vi "主程序.vi"() -> ()   [LabVIEW 2012]
uses:
  <vilib>/Utility/miscctls.llb/LVRGBAColorTypeDef.ctl
  <vilib>/addons/control/pid/pid.llb/PID (DBL).vi
  <vilib>/addons/control/pid/NI_PID_pid.lvlib
  <vilib>/picture/3D Picture Control/NI_3D Picture Control.lvlib
panel:
  out "摆臂角度":dbl(graph)=-1.40625
  out "旋转臂角度":cluster{"旋转臂测量角度 3":dbl, dbl}(graph)={"旋转臂测量角度 3"=-61.25, -2.1437500000000003}
  out "输出电压":dbl(graph)=0.6637500000000003
  in  "输出电压1":dbl(graph)=0.6637500000000003
  out "三维图片":refnum<vi>(3d-picture)
  out "程序状态":bool=TRUE
  in  "继续按钮":bool
  in  "暂停按钮":bool
  out "摆臂角度输出 2":dbl=898.59375
  out "摆臂角度输出":dbl=178.59375
  out "摆臂角度1":dbl(graph)=-1.40625
  out "旋转臂角度1":cluster{"旋转臂测量角度 3":dbl, dbl}(graph)={"旋转臂测量角度 3"=-61.25, -2.1437500000000003}
  in  "副控制器PID参数":T1={"比例系数(Kc)"=0.9, "积分系数(Ti,min)"=0.0, "微分时间(Td/min)"=0.001}
  in  "主控制器PID参数":T1={"比例系数(Kc)"=0.035, "积分系数(Ti,min)"=0.0, "微分时间(Td/min)"=0.009}
  in  "?":bool=TRUE
  in  "副控制器设定值":dbl
  in  "K1":dbl=0.02
  in  "K2":dbl=-0.0
  in  "副控制器控制周期":u32=5
  out "output":dbl=-2.1437500000000003 format="%.2f"
  in  "停止":bool
  in  "主控制器控制周期":u32=15
  out "旋转臂测量角度 3":dbl=-61.25
  in  "主控制器设定值":dbl format="%.2f"
  # "一阶倒立摆串级PID控制\n测控技术与仪器                       1502班                                刘芳扬"
  # "副控制器系数"
  # "三维视图"
  # "测量显示"
  # "ms"
  # "控制方式"
  # "单回路"
  # "串级"
  # "主控制器系数"
  # "启停设置"
  # "ms"
  # "起摆系数"
  # "程序停止"
  # "程序暂停"
  # "程序继续"
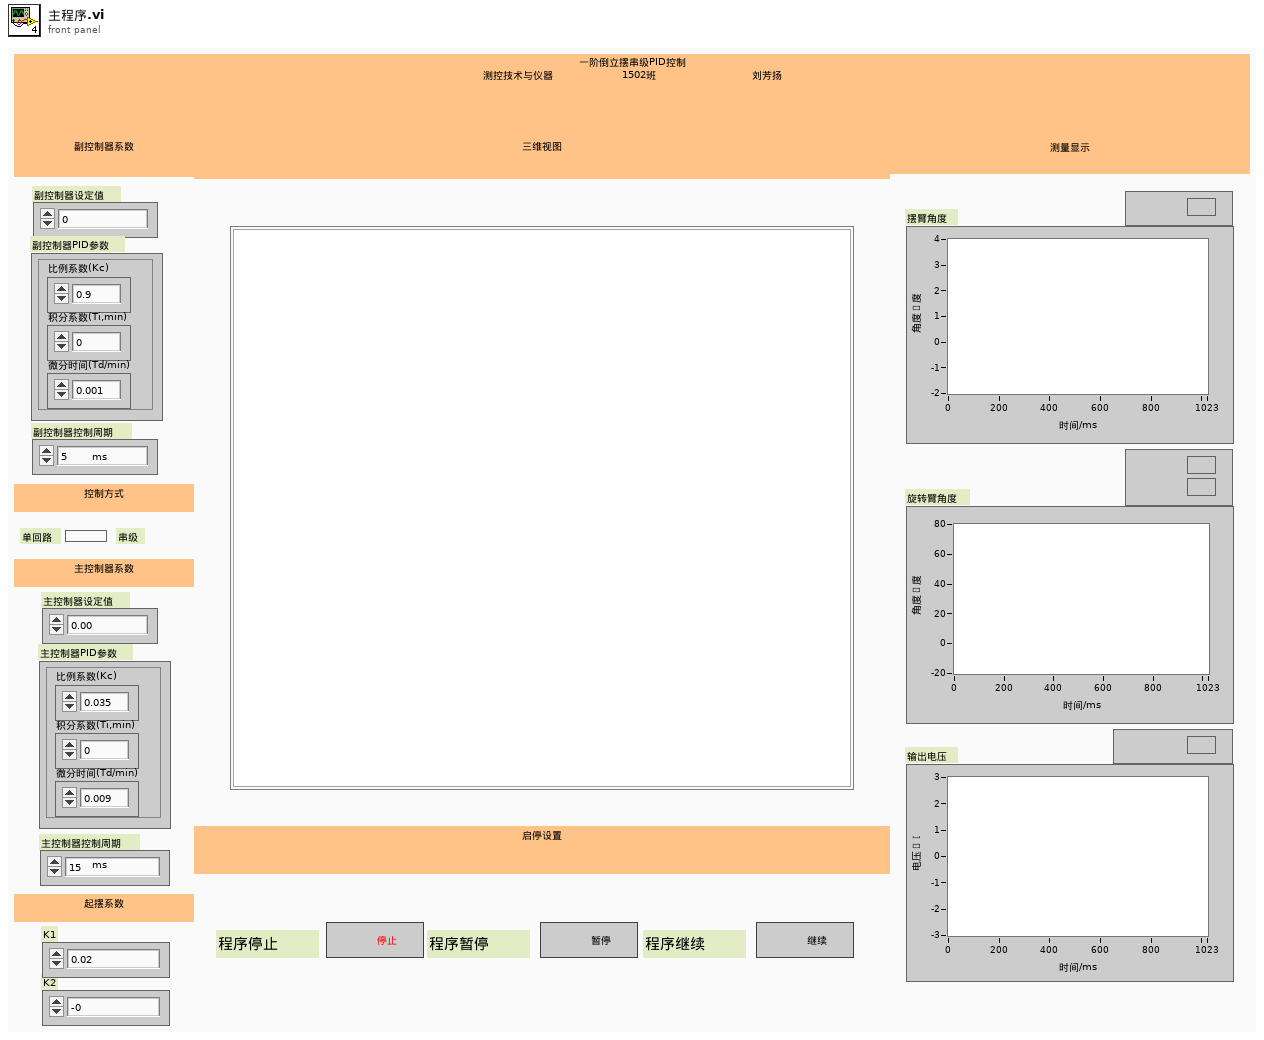
[diagram p1: front panel]
types:
  T1 = cluster{"比例系数(Kc)":dbl, "积分系数(Ti,min)":dbl, "微分时间(Td/min)":dbl}
  T2 = typedef "LVRGBAColorTypeDef.ctl" = cluster{"Red":sgl, "Green":sgl, "Blue":sgl, "Alpha":sgl}
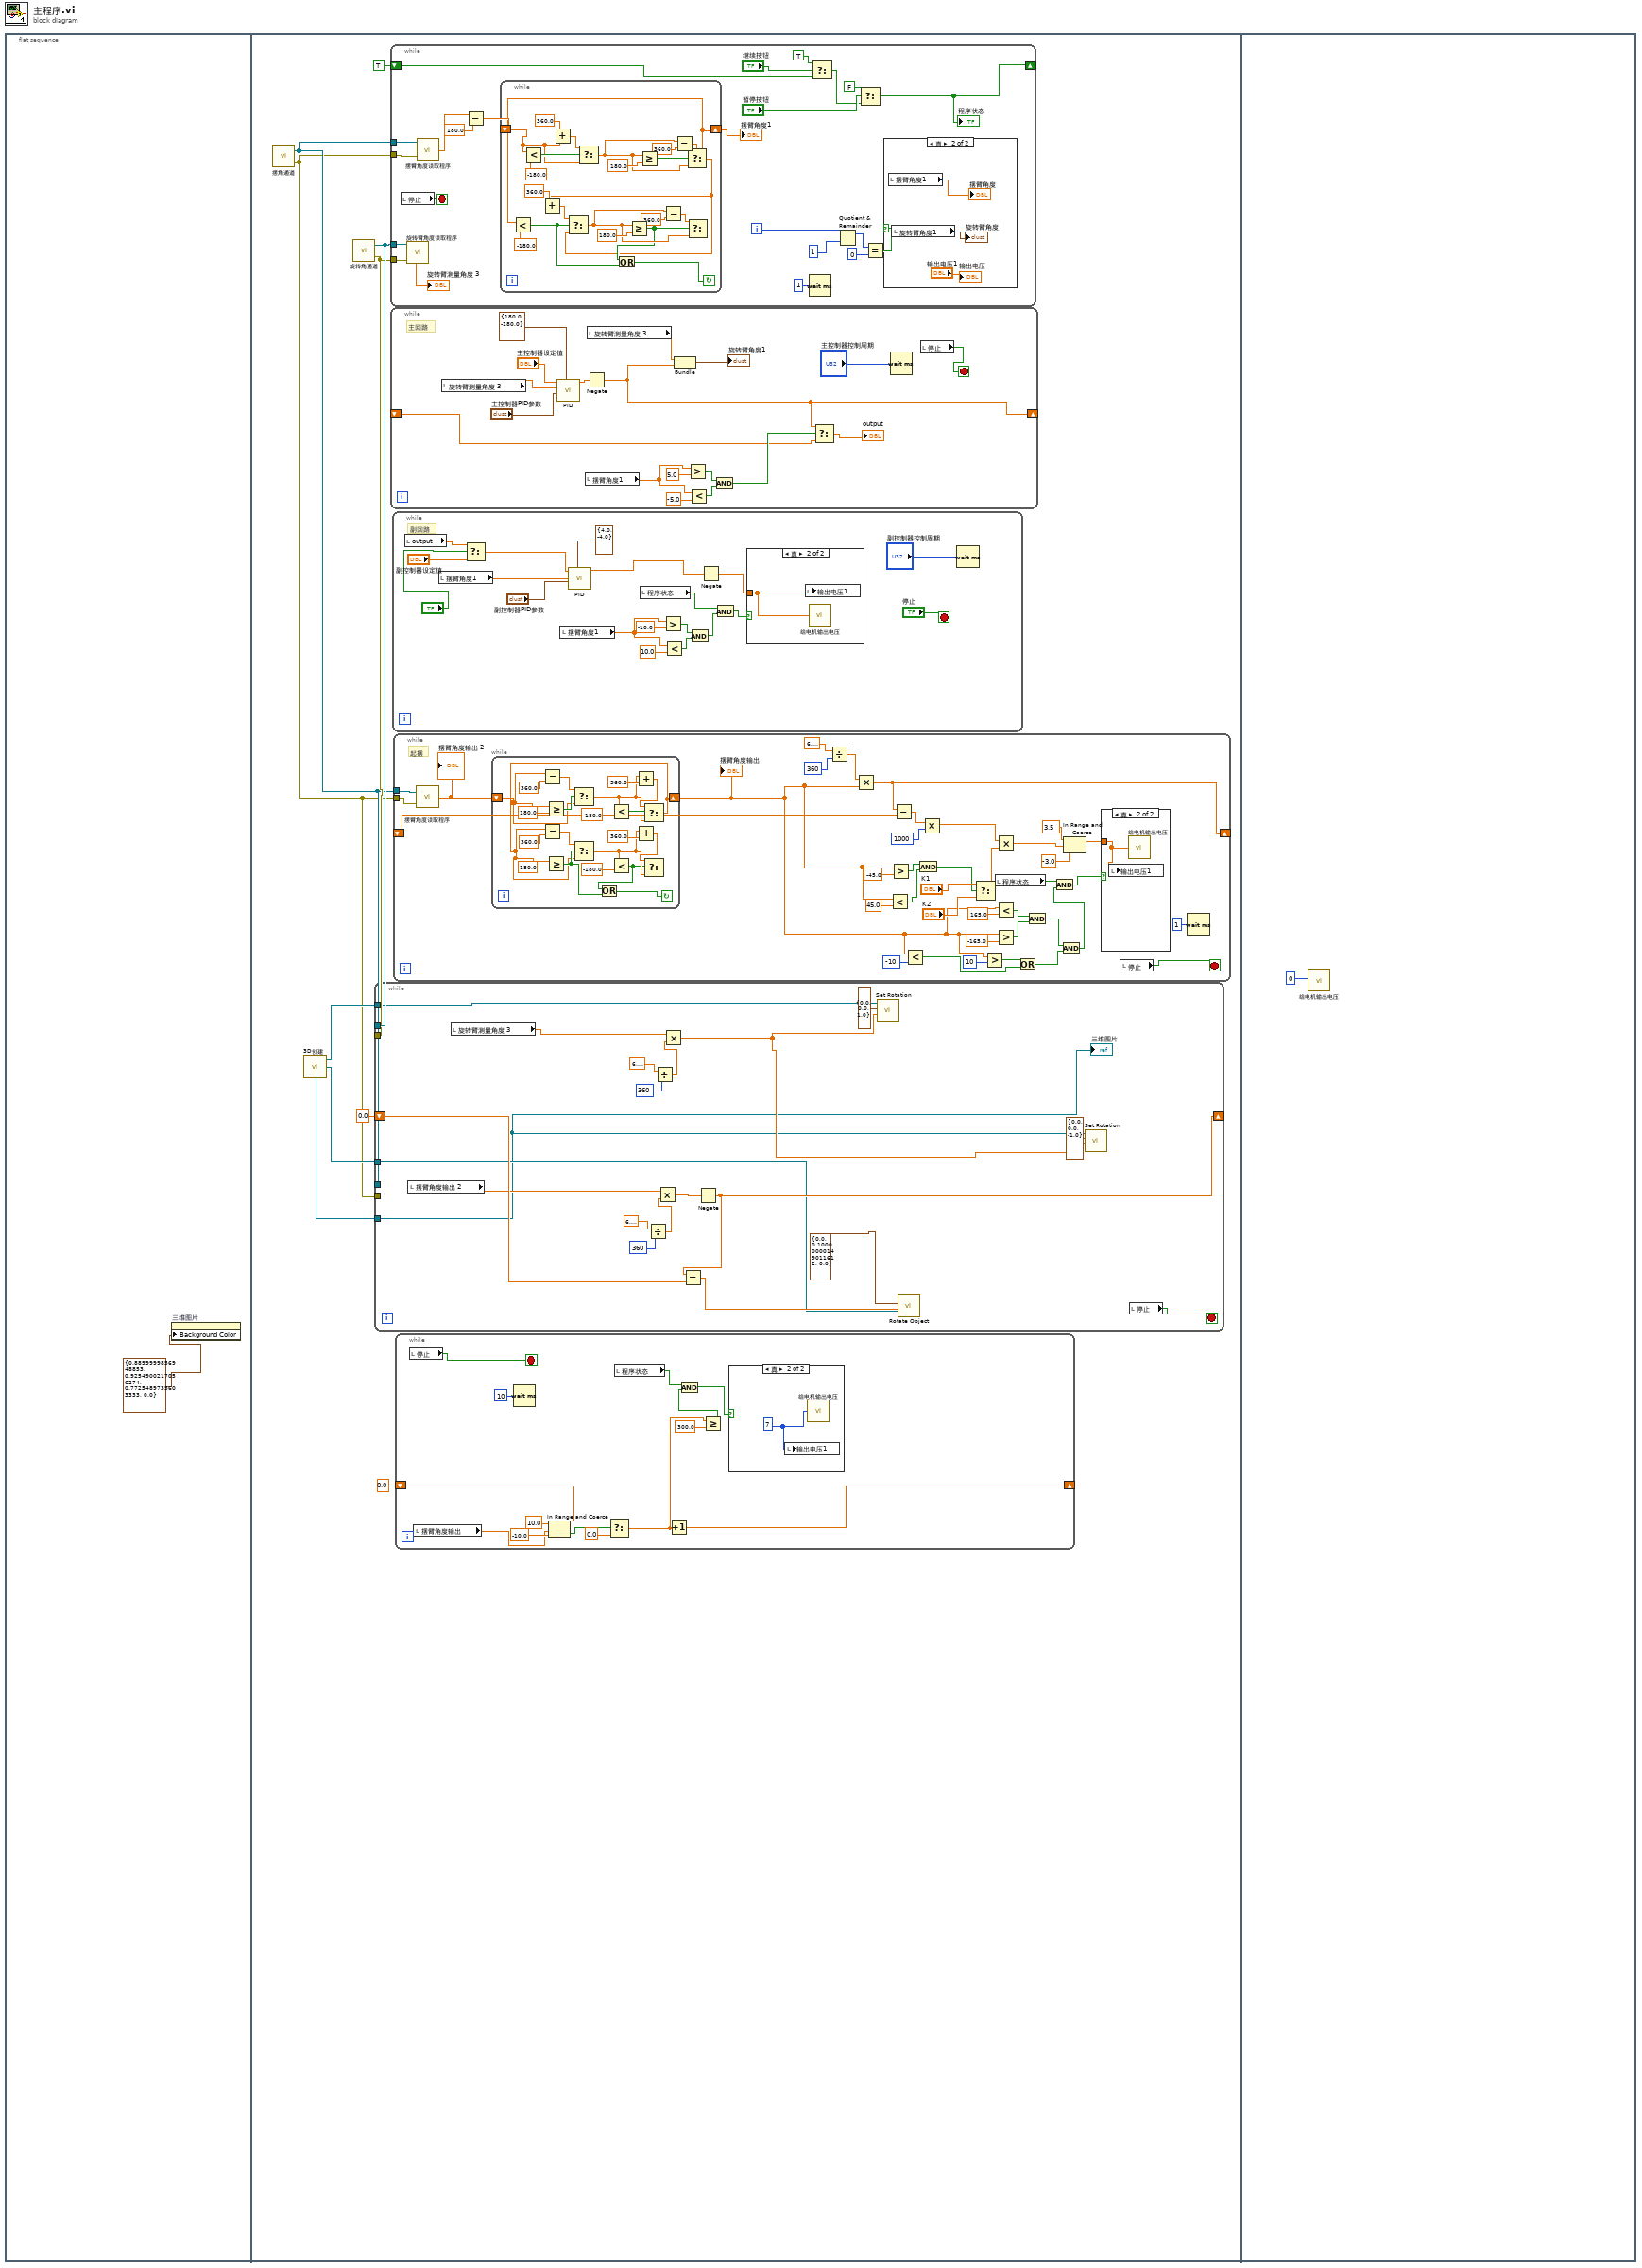
[diagram p0: block diagram]
diagram:
  n1 = flat-sequence {
    frame #0 {
      n2 = property on="三维图片" class="SceneGraphDisp (严格)"("Background Color"=T2 {"Red"=0.89, "Green"=0.92549, "Blue"=0.772549, "Alpha"=0.0} ("背景色")) -> ()  [unwired: 2 in, 2 out]
    }
    frame #1 {
      n3 = call "摆角通道.vi"() -> ("error out"=w5:errorcluster, "task out"=w6:refnum<k21>)  [unwired: 2 in]
      n4 = call "3D创建.vi"() -> ("旋转臂"=w9:refnum<vi>, "摆臂"=w10:refnum<vi>, "底座"=w11:refnum<vi>)
      n5 = call "旋转角通道.vi"() -> ("error out"=w7:errorcluster, "task out"=w8:refnum<k21>)  [unwired: 2 in]
      n6 = while {
        tunnel: w11 -> [w29]
        tunnel: w10 -> [w28]
        tunnel: w9 -> [w27]
        shift-right: [w33] -> _
        shift-left: 0.0 -> [w34]
        tunnel: w8 -> [_]
        tunnel: w7 -> [_]
        tunnel: w6 -> [_]
        tunnel: w5 -> [_]
        stop <- w32 stop-if-true
        n7 = local read "摆臂角度输出 2"() -> (w30:dbl)
        n8 = local read "旋转臂测量角度 3"() -> (w31:dbl)
        n9 = Divide(x=6.283185307179586, y=360) -> (x/y=w41:dbl)
        n10 = Divide(x=6.283185307179586, y=360) -> (x/y=w44:dbl)
        n11 = Multiply(x=w30, y=w41) -> (x*y=w38:dbl)
        n12 = Multiply(x=w31, y=w44) -> (x*y=w35:dbl)
        n13 = Negate(x=w38) -> (-x=w33:dbl)
        n14 = Subtract(x=w33, y=w34) -> (x-y=w37:dbl)
        n15 = call <vilib>:"Set Rotation.vi"("Angle"=w35, "Axis"=cluster{"X":sgl, "Y":sgl, "Z":sgl} {"X"=0.0, "Y"=0.0, "Z"=1.0}, "Scene Object"=w29) -> ()  [unwired: 7 in, 2 out]
        n16 = call <vilib>:"Rotate Object.vi"("Angle"=w37, "Axis"=cluster{"X":sgl, "Y":sgl, "Z":sgl} {"X"=0.0, "Y"=0.1, "Z"=0.0}, "Scene.Object In"=w28) -> ()  [unwired: 7 in, 2 out]
        n17 = call <vilib>:"Set Rotation.vi"("Angle"=w35, "Axis"=cluster{"X":sgl, "Y":sgl, "Z":sgl} {"X"=0.0, "Y"=0.0, "Z"=-1.0}, "Scene Object"=w27) -> ()  [unwired: 7 in, 2 out]
        n18 = local read "停止"() -> (w32:bool)
        "三维图片" <- w27
      }
      n19 = while {
        tunnel: w5 -> [w160]
        tunnel: w6 -> [w161]
        tunnel: w8 -> [w167]
        tunnel: w7 -> [w166]
        shift-right: [w152] -> _
        shift-left: TRUE -> [w151]
        i -> [w150]
        stop <- w158 stop-if-true
        n20 = local read "停止"() -> (w158:bool)
        n21 = call "旋转臂角度读取程序.vi"("error out"=w166, "task out 2"=w167) -> ("旋转臂测量角度"=→"旋转臂测量角度 3":dbl)
        n22 = call "摆臂角度读取程序.vi"("error in"=w160, "task/channels in"=w161) -> ("摆臂角度输出"=w159:dbl)
        n23 = Subtract(x=w159, y=180.0) -> (x-y=w163:dbl)
        n24 = while {
          shift-right: [w173] -> w162
          shift-left: w163 -> [w172]
          stop <- w174 continue-if-true
          n25 = Less?(x=w172, y=-180.0) -> (x < y?=w191:bool)
          n26 = Add(x=w172, y=360.0) -> (x+y=w189:dbl)
          n27 = Select(t=w189, s=w191, f=w172) -> (s? t:f=w184:dbl)
          n28 = Greater Or Equal?(x=w184, y=180.0) -> (x >= y?=w188:bool)
          n29 = Subtract(x=w184, y=360.0) -> (x-y=w185:dbl)
          n30 = Select(t=w185, s=w188, f=w184) -> (s? t:f=w173:dbl)
          n31 = Less?(x=w173, y=-180.0) -> (x < y?=w175:bool)
          n32 = Add(x=w173, y=360.0) -> (x+y=w181:dbl)
          n33 = Select(t=w181, s=w175, f=w173) -> (s? t:f=w177:dbl)
          n34 = Greater Or Equal?(x=w177, y=180.0) -> (x >= y?=w176:bool)
          n35 = Or(x=w176, y=w175) -> (x .or. y?=w174:bool)
          n36 = Subtract(x=w177, y=360.0) -> (x-y=w178:dbl)
          n37 = Select(t=w178, s=w176, f=w177) -> ()  [unwired: 1 out]
        }
        "摆臂角度1" <- w162
        n38 = Wait (ms)(milliseconds to wait=u32 1 ("等待时间（毫秒）")) -> ()  [unwired: 1 out]
        n39 = Select(t=TRUE, s="继续按钮", f=w151) -> (s? t:f=w155:bool)
        n40 = Quotient & Remainder(x=w150, y=1) -> (x-y*floor(x/y)=w146:i32)  [unwired: 1 out]
        n41 = Select(t=FALSE, s="暂停按钮", f=w155) -> (s? t:f=w152:bool)
        "程序状态" <- w152
        n42 = Equal?(x=w146, y=0) -> (x = y?=w147:bool)
        n43 = case shown="真" w147 {
          frame False {
          }
          frame True {
            n44 = local read "摆臂角度1"() -> (→"摆臂角度":dbl)
            n45 = local read "旋转臂角度1"() -> (→"旋转臂角度":cluster{"旋转臂测量角度 3":dbl, dbl})
            "输出电压" <- "输出电压1"
          }
        }
      }
      n46 = while {
        shift-right: [w133] -> _
        shift-left: _ -> [w132]
        stop <- w128 stop-if-true
        # "主回路"
        n47 = local read "旋转臂测量角度 3"() -> (w145:dbl)
        n48 = call-poly <vilib>:"PID.vi"("output range"=cluster{"output high":dbl, "output low":dbl} {"output high"=180.0, "output low"=-180.0}, "PID gains"="主控制器PID参数", "process variable"=w145, "setpoint"="主控制器设定值") -> ("output"=w140:dbl)  [unwired: 6 in, 1 out]
        n49 = local read "摆臂角度1"() -> (w135:dbl)
        n50 = Negate(x=w140) -> (-x=w133:dbl)
        n51 = local read "旋转臂测量角度 3"() -> (w142:dbl)
        n52 = Bundle("旋转臂测量角度 3"=w142, w133) -> (→"旋转臂角度1":cluster{"旋转臂测量角度 3":dbl, dbl})  [unwired: 1 in]
        n53 = Greater?(x=w135, y=5.0) -> (0:w136:bool)
        n54 = Less?(x=w135, y=-5.0) -> (x < y?=w137:bool)
        n55 = And(x=w136, y=w137) -> (x .and. y?=w134:bool)
        n56 = Select(t=w133, s=w134, f=w132) -> (s? t:f=→"output":dbl)
        n57 = Wait (ms)(milliseconds to wait="主控制器控制周期") -> ()  [unwired: 1 out]
        n58 = local read "停止"() -> (w128:bool)
      }
      n59 = while {
        stop <- "停止" stop-if-true
        # "副回路"
        n60 = local read "output"() -> (w115:dbl)
        n61 = local read "摆臂角度1"() -> (w123:dbl)
        n62 = Select(t=w115, s="?", f="副控制器设定值") -> (s? t:f=w112:dbl)
        n63 = local read "摆臂角度1"() -> (w117:dbl)
        n64 = call-poly <vilib>:"PID.vi"("output range"=cluster{"output high":dbl, "output low":dbl} {"output high"=4.0, "output low"=-4.0} ("内回路上下限"), "PID gains"="副控制器PID参数", "process variable"=w123, "setpoint"=w112) -> ("output"=w116:dbl)  [unwired: 6 in, 1 out]
        n65 = local read "程序状态"() -> (w108:bool)
        n66 = Greater?(x=w117, y=-10.0) -> (0:w118:bool)
        n67 = Less?(x=w117, y=10.0) -> (x < y?=w119:bool)
        n68 = And(x=w118, y=w119) -> (x .and. y?=w110:bool)
        n69 = Negate(x=w116) -> (-x=w122:dbl)
        n70 = And(x=w108, y=w110) -> (x .and. y?=w109:bool)
        n71 = case shown="真" w109 {
          tunnel: w122 -> [_ w127]
          frame False {
          }
          frame True {
            n72 = local write "输出电压1"(w127) -> ()
            n73 = call "给电机输出电压.vi"("电压输入"=w127) -> ()
          }
        }
        n74 = Wait (ms)(milliseconds to wait="副控制器控制周期") -> ()  [unwired: 1 out]
      }
      n75 = while {
        tunnel: w6 -> [w85]
        shift-right: [w80] -> _
        shift-left: _ -> [w79]
        tunnel: w5 -> [w64]
        stop <- w59 stop-if-true
        # "起摆"
        n76 = call "摆臂角度读取程序.vi"("error in"=w64, "task/channels in"=w85) -> ("摆臂角度输出"=w63:dbl)
        "摆臂角度输出 2" <- w63
        n77 = while {
          shift-right: [w86] -> w55
          shift-left: w63 -> [w100]
          stop <- w87 continue-if-true
          n78 = Subtract(x=w100, y=360.0) -> (x-y=w103:dbl)
          n79 = Greater Or Equal?(x=w100, y=180.0) -> (x >= y?=w105:bool)
          n80 = Select(t=w103, s=w105, f=w100) -> (s? t:f=w97:dbl)
          n81 = Less?(x=w97, y=-180.0) -> (x < y?=w101:bool)
          n82 = Add(x=w97, y=360.0) -> (x+y=w99:dbl)
          n83 = Select(t=w99, s=w101, f=w97) -> (s? t:f=w86:dbl)
          n84 = Subtract(x=w86, y=360.0) -> (x-y=w94:dbl)
          n85 = Greater Or Equal?(x=w86, y=180.0) -> (x >= y?=w88:bool)
          n86 = Select(t=w94, s=w88, f=w86) -> (s? t:f=w90:dbl)
          n87 = Less?(x=w90, y=-180.0) -> (x < y?=w89:bool)
          n88 = Or(x=w89, y=w88) -> (x .or. y?=w87:bool)
          n89 = Add(x=w90, y=360.0) -> (x+y=w92:dbl)
          n90 = Select(t=w92, s=w89, f=w90) -> ()  [unwired: 1 out]
        }
        "摆臂角度输出" <- w55
        n91 = Divide(x=6.283185307179586, y=360) -> (x/y=w82:dbl)
        n92 = Multiply(x=w82, y=w55) -> (x*y=w80:dbl)
        n93 = Less?(x=w55, y=45.0) -> (x < y?=w67:bool)
        n94 = Greater?(x=w55, y=-45.0) -> (0:w68:bool)
        n95 = Subtract(x=w80, y=w79) -> (x-y=w78:dbl)
        n96 = Less?(x=w55, y=-10) -> (x < y?=w54:bool)
        n97 = And(x=w68, y=w67) -> (x .and. y?=w66:bool)
        n98 = Multiply(x=w78, y=1000) -> (x*y=w76:dbl)
        n99 = Select(t="K1", s=w66, f="K2") -> (s? t:f=w65:dbl)
        n100 = Greater?(x=w55, y=10) -> (0:w57:bool)
        n101 = Multiply(x=w76, y=w65) -> (x*y=w75:dbl)
        n102 = local read "程序状态"() -> (w49:bool)
        n103 = Less?(x=w55, y=165.0) -> (x < y?=w61:bool)
        n104 = Greater?(x=w55, y=-165.0) -> (0:w47:bool)
        n105 = Or(x=w57, y=w54) -> (x .or. y?=w53:bool)
        n106 = And(x=w61, y=w47) -> (x .and. y?=w52:bool)
        n107 = And(x=w52, y=w53) -> (x .and. y?=w50:bool)
        n108 = And(x=w49, y=w50) -> (x .and. y?=w51:bool)
        n109 = In Range and Coerce(upper limit=3.5 ("上限"), x=w75, lower limit=-3.0 ("下限")) -> (coerced(x)=w72:dbl)  [unwired: 1 out]
        n110 = case shown="真" w51 {
          tunnel: w72 -> [_ w107]
          frame False {
          }
          frame True {
            n111 = local write "输出电压1"(w107) -> ()
            n112 = call "给电机输出电压.vi"("电压输入"=w107) -> ()
          }
        }
        n113 = local read "停止"() -> (w59:bool)
        n114 = Wait (ms)(milliseconds to wait=u32 1 ("等待时间（毫秒）")) -> ()  [unwired: 1 out]
      }
      n115 = while {
        shift-right: [w19] -> _
        shift-left: 0.0 ("f") -> [w21]
        stop <- w20 stop-if-true
        n116 = local read "停止"() -> (w20:bool)
        n117 = local read "摆臂角度输出"() -> (w15:dbl)
        n118 = Wait (ms)(milliseconds to wait=u32 10 ("等待时间（毫秒）")) -> ()  [unwired: 1 out]
        n119 = In Range and Coerce(upper limit=10.0 ("上限"), x=w15, lower limit=-10.0 ("下限")) -> (In Range?=w23:bool)  [unwired: 1 out]
        n120 = Select(t=w21, s=w23, f=0.0) -> (s? t:f=w16:dbl)
        n121 = local read "程序状态"() -> (w12:bool)
        n122 = Increment(x=w16) -> (x+1=w19:dbl)
        n123 = Greater Or Equal?(x=w16, y=300.0) -> (x >= y?=w13:bool)
        n124 = And(x=w12, y=w13) -> (x .and. y?=w14:bool)
        n125 = case shown="真" w14 {
          frame False {
          }
          frame True {
            w26 = 7
            n126 = local write "输出电压1"(w26) -> ()
            n127 = call "给电机输出电压.vi"("电压输入"=w26) -> ()
          }
        }
      }
    }
    frame #2 {
      n128 = call "给电机输出电压.vi"("电压输入"=0) -> ()
    }
  }
